vi "Config - Update.vi"(8 "error in (no error)":errorcluster, 11 "View Model":T1) -> (0 "error out":errorcluster, 3 "View Model":T1)   [LabVIEW 2017]
doc: "Reads DB record from Configuration database."
uses:
  View Model/Controls/View Model.ctl
  View Model/Controls/Shared Model.ctl
  Error/Controls/Error Model.ctl
  Error/Controls/Error Event.ctl
  Error/Controls/Error Type.ctl
  Controls/Config DB Model.ctl
  Controls/Config DB Command.ctl
  Controls/Config DB Record.ctl
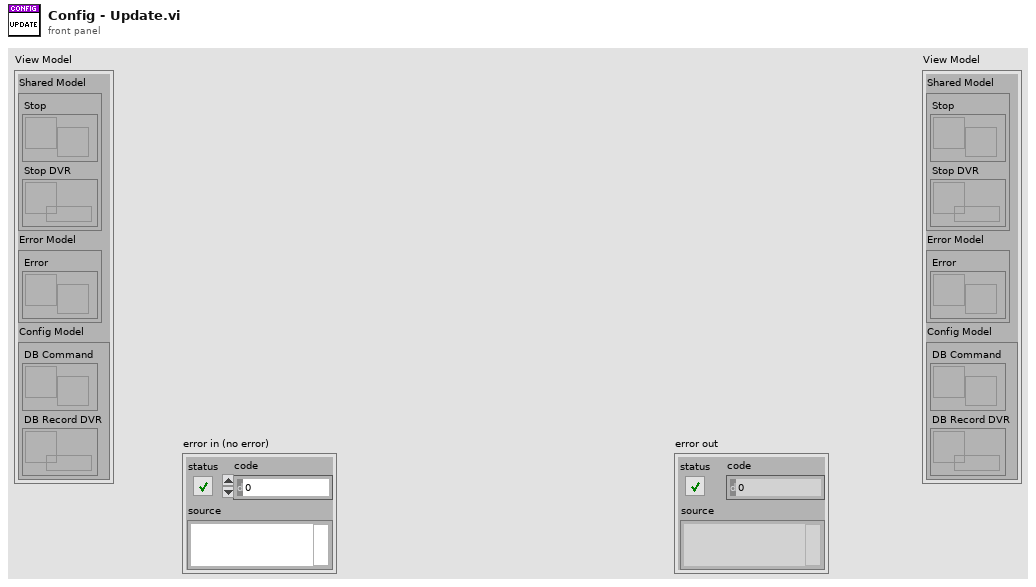
[diagram p1: front panel]
types:
  T1 = typedef "View Model.ctl" = cluster{"Shared Model":T2, "Error Model":T3, "Config Model":T4}
  T2 = typedef "Shared Model.ctl" = cluster{"Stop":refnum<user-event>, "Stop DVR":refnum<data-value>}
  T3 = typedef "Error Model.ctl" = cluster{"Error":refnum<user-event>}
  T4 = typedef "Config DB Model.ctl" = cluster{"DB Command":refnum<user-event>, "DB Record DVR":refnum<data-value>}
  T5 = enum16{"open", "replace", "create", "open or create", "replace or create", "replace or create with confirmation"}
  T6 = typedef "Config DB Record.ctl" = cluster{"Door Open":dbl, "Door Close":dbl, "Travel Time":dbl, "Inactivity Time":dbl}
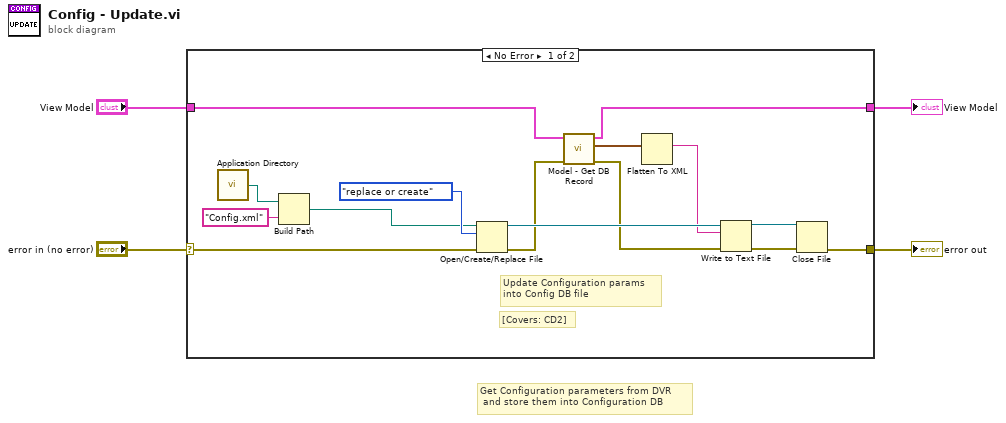
[diagram p0: block diagram]
diagram:
  # "Get Configuration parameters from DVR\n and store them into Configuration DB"
  n1 = case shown="No Error" "error in (no error)" {
    selector: "error in (no error)" -> [w15 w20]
    tunnel: "View Model" -> [w11 w21]
    tunnel: [w6 w21] -> w2
    tunnel: [w5 w20] -> w1
    frame No Error {
      # "[Covers: CD2]"
      # "Update Configuration params\ninto Config DB file"
      n2 = call <vilib>:"Application Directory.vi"() -> ("Application Directory"=w19:path)
      n3 = Build Path(base path=w19, name or relative path="Config.xml") -> (appended path=w16:path)
      n4 = Open/Create/Replace File(file path (use dialog)=w16, error in=w15, operation (0:open)=T5."replace or create") -> (refnum out=w14:refnum<file>, error out=w9:errorcluster)  [unwired: 3 in, 1 out]
      n5 = call "Model - Get DB Record.vi"("error in (no error)"=w9, "View Model"=w11) -> ("error out"=w8:errorcluster, "DB Record"=w10:T6, "View Model"=w6:T1)  [unwired: 7 in]
      n6 = Flatten To XML(anything=w10) -> (xml string=w7:string)
      n7 = Write to Text File(file (use dialog)=w14, text=w7, error in=w8) -> (refnum out=w13:refnum<file>, error out=w12:errorcluster)  [unwired: 1 in, 1 out]
      n8 = Close File(refnum=w13, error in=w12) -> (error out=w5:errorcluster)  [unwired: 1 out]
    }
    frame Error {
    }
  }
  "error out" <- w1
  "View Model" <- w2
